vi "Check_Aero_Tunnel_on_Server.vi"(1 "Current Time":dbl format="%.2f", 2 "Ch Names":string[](array[string]), 3 "Values":dbl[](array[numeric]) format="%.2f") -> ()   [LabVIEW 2010]
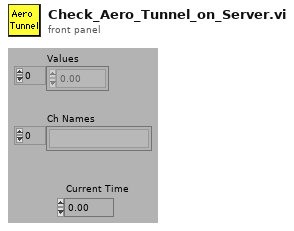
[diagram p1: front panel]
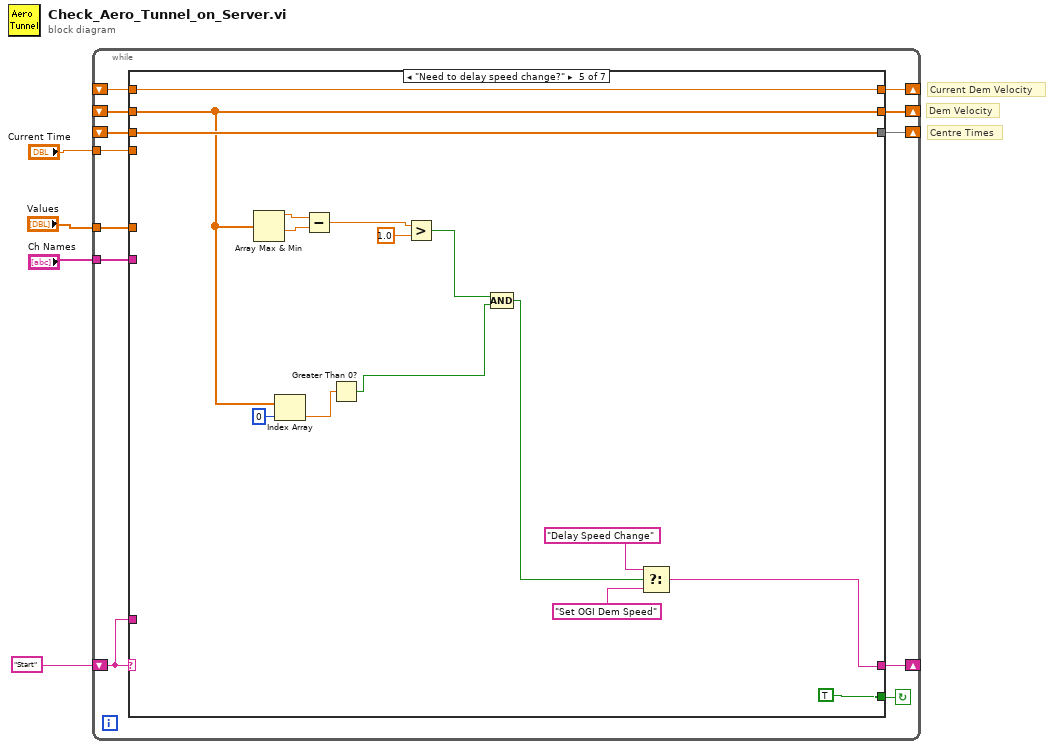
[diagram p0: block diagram]
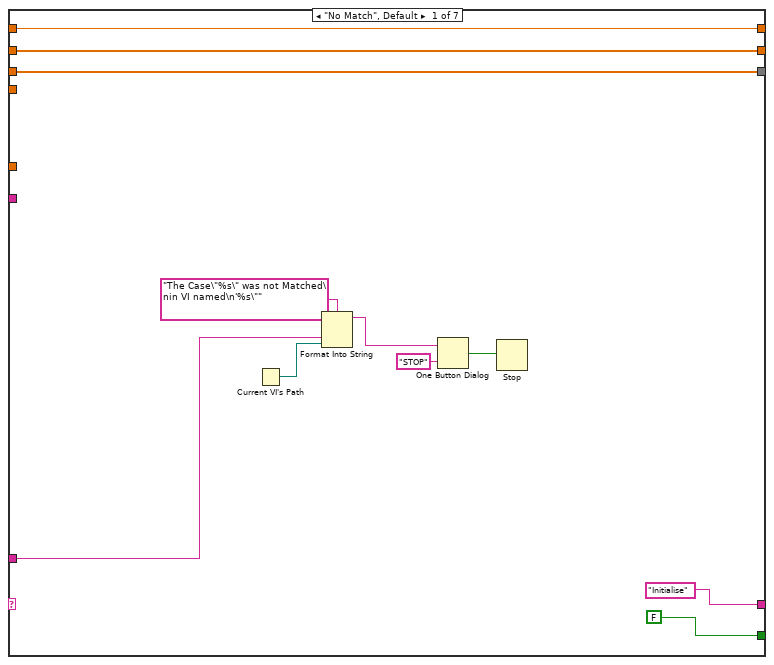
[diagram p2: hidden frame]
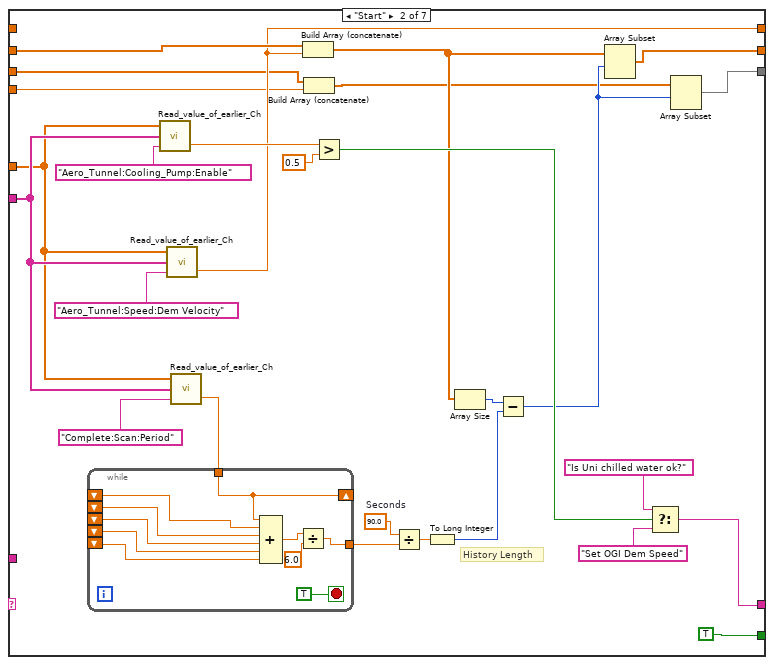
[diagram p3: hidden frame]
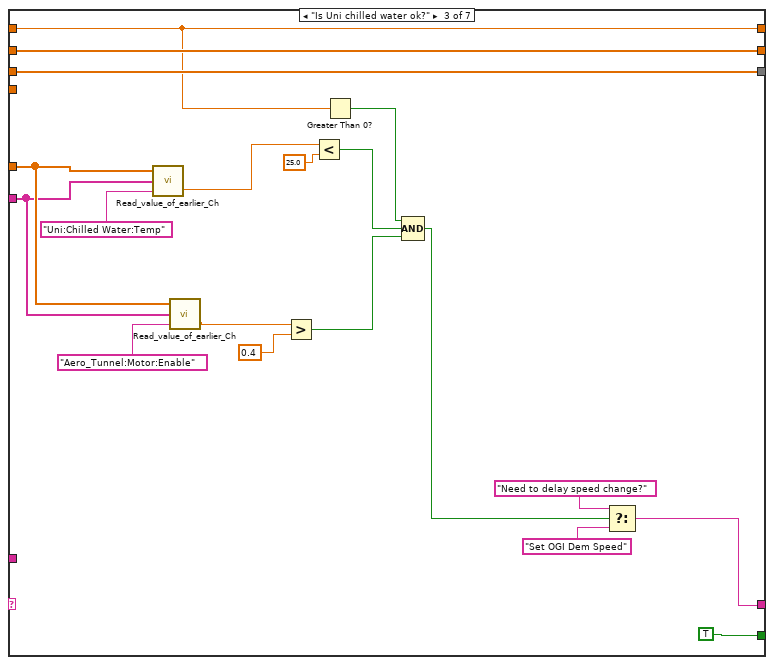
[diagram p4: hidden frame]
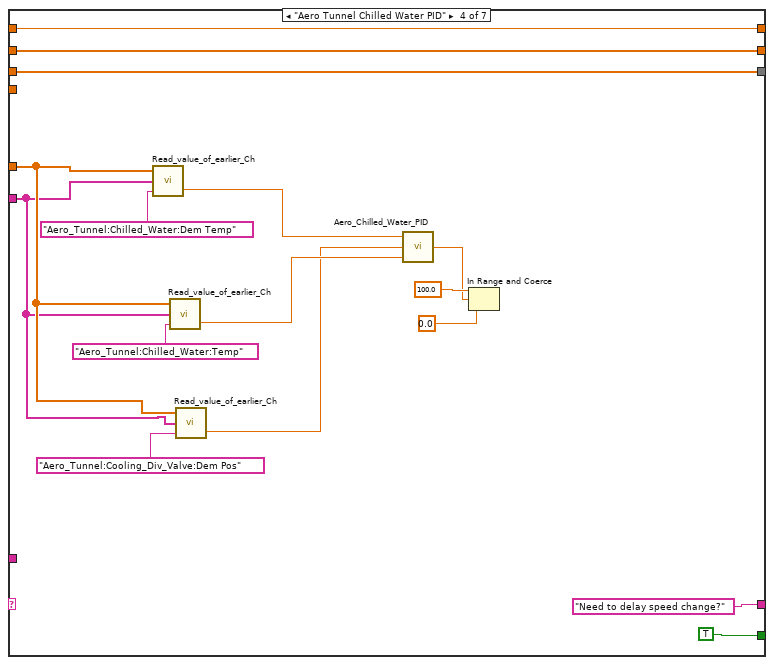
[diagram p5: hidden frame]
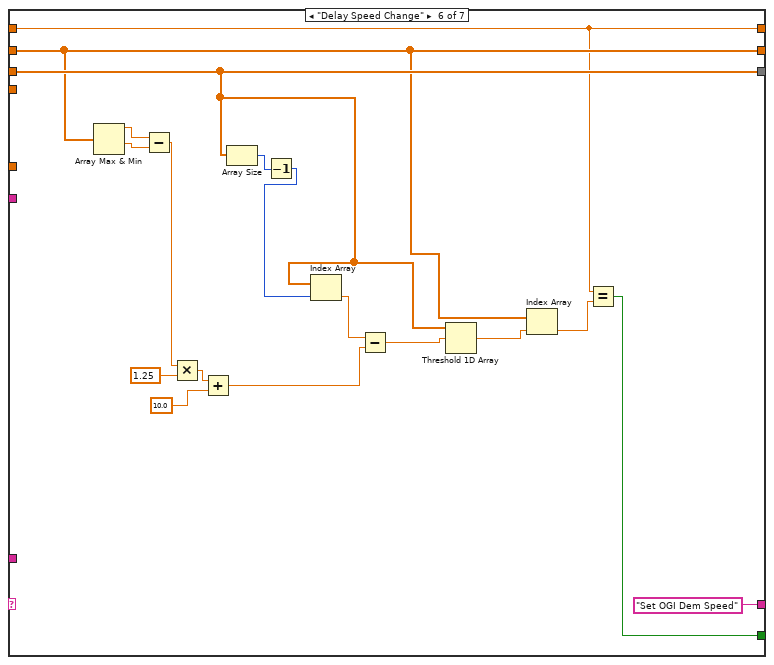
[diagram p6: hidden frame]
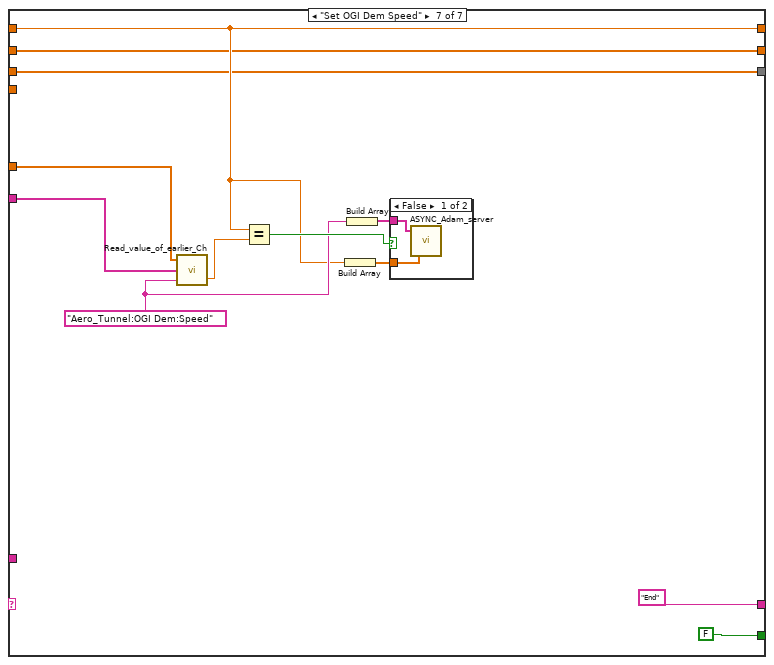
[diagram p7: hidden frame]
diagram:
  # "Dem Velocity"
  # "Centre Times"
  # "Current Dem Velocity"
  n1 = while {
    shift-left: "Start" -> [w14]
    shift-right: [w15] -> _
    tunnel: "Values" -> [w13]
    tunnel: "Ch Names" -> [w12]
    shift-right: [w11] -> _
    shift-left: _ -> [w10]
    shift-right: [w8] -> _
    shift-left: _ -> [w9]
    shift-right: [w5] -> _
    shift-left: _ -> [w6]
    tunnel: "Current Time" -> [w7]
    stop <- w16 continue-if-true
    n2 = case shown="\"Need to delay speed change?\"" w14 {
      tunnel: [FALSE TRUE TRUE TRUE TRUE w117 FALSE] -> w16
      tunnel: ["Initialise" w47 w78 "Need to delay speed change?" ("t") w113 "Set OGI Dem Speed" "End"] -> w15
      tunnel: w14 -> [w22 _ _ _ _ _ _]
      tunnel: w13 -> [_ w43 w73 w87 _ _ w143]
      tunnel: w12 -> [_ w44 w72 w86 _ _ w142]
      tunnel: [w19 w38 w67 w94 w107 w118 w136] -> w11
      tunnel: w10 -> [w19 _ w67 w94 w107 w118 w136]
      tunnel: w9 -> [w18 w39 w77 w97 w105 w119 w135]
      tunnel: [w18 w34 w77 w97 w105 w119 w135] -> w8
      tunnel: w7 -> [_ w31 _ _ _ _ _]
      tunnel: w6 -> [w17 w30 w76 w96 w112 w120 w134]
      tunnel: [w17 w28 w76 w96 w112 w120 w134] -> w5
      frame "No Match", Default {
        n3 = Current VI's Path() -> (path=w21:path)
        n4 = Format Into String(format string="The Case\"%s\" was not Matched\nin VI named\n'%s\"" ("Format String"), w22, w21) -> (resulting string=w25:string)  [unwired: 2 in, 1 out]
        n5 = One Button Dialog(message=w25, button name ("OK")="STOP") -> (true=w23:bool)
        n6 = Stop(stop? (T)=w23) -> ()
      }
      frame "Start" {
        w40 = 90.0  # Seconds
        # "History Length"
        n7 = call "Read_value_of_earlier_Ch.vi"("Desired Ch to Read"="Aero_Tunnel:Cooling_Pump:Enable", "Ch names"=w44, "Present scan array"=w43) -> ("Value"=w51:dbl)  [unwired: 1 in, 1 out]
        n8 = call "Read_value_of_earlier_Ch.vi"("Desired Ch to Read"="Aero_Tunnel:Speed:Dem Velocity", "Ch names"=w44, "Present scan array"=w43) -> ("Value"=w38:dbl)  [unwired: 1 in, 1 out]
        n9 = call "Read_value_of_earlier_Ch.vi"("Desired Ch to Read"="Complete:Scan:Period", "Ch names"=w44, "Present scan array"=w43) -> ("Value"=w42:dbl)  [unwired: 1 in, 1 out]
        n10 = while {
          shift-right: [w64] -> _
          shift-left: _ -> [w63]
          tunnel: w42 -> [w64]
          shift-left: _ -> [w62]
          shift-left: _ -> [w61]
          shift-left: _ -> [w60]
          shift-left: _ -> [w59]
          tunnel: [w55] -> w41
          stop <- TRUE stop-if-true
          n11 = Compound Arithmetic op=ADD(w64, w63, w62, w61, w60, w59) -> (w57:dbl)
          n12 = Divide(x=w57, y=6.0) -> (x/y=w55:dbl)
        }
        n13 = Build Array (concatenate)(w39, w38) -> (w32:dbl[])
        n14 = Build Array (concatenate)(w30, w31) -> (w29:dbl[])
        n15 = Greater?(x=w51, y=0.5) -> (0:w49:bool)
        n16 = Divide(x=w40, y=w41) -> (x/y=w36:dbl)
        n17 = To Long Integer(number=w36) -> (32bit integer=w35:i32)
        n18 = Array Size(array=w32) -> (size(s)=w37:i32)
        n19 = Subtract(x=w37, y=w35) -> (x-y=w33:i32)
        n20 = Array Subset(array=w32, index=w33) -> (w34:dbl[])  [unwired: 1 in]
        n21 = Select(t="Is Uni chilled water ok?", s=w49, f="Set OGI Dem Speed") -> (s? t:f=w47:string)
        n22 = Array Subset(array=w29, index=w33) -> (w28:dbl[])  [unwired: 1 in]
      }
      frame "Is Uni chilled water ok?" {
        n23 = call "Read_value_of_earlier_Ch.vi"("Desired Ch to Read"="Uni:Chilled Water:Temp", "Ch names"=w72, "Present scan array"=w73) -> ("Value"=w81:dbl)  [unwired: 1 in, 1 out]
        n24 = call "Read_value_of_earlier_Ch.vi"("Desired Ch to Read"="Aero_Tunnel:Motor:Enable", "Ch names"=w72, "Present scan array"=w73) -> ("Value"=w70:dbl)  [unwired: 1 in, 1 out]
        n25 = Greater?(x=w70, y=0.4) -> (0:w68:bool)
        n26 = Less?(x=w81, y=25.0) -> (x < y?=w69:bool)
        n27 = Greater Than 0?(x=w67) -> (x > 0?=w66:bool)
        n28 = Compound Arithmetic op=AND(w66, w69, w68) -> (w65:bool)
        n29 = Select(t="Need to delay speed change?", s=w65, f="Set OGI Dem Speed") -> (s? t:f=w78:string)
      }
      frame "Aero Tunnel Chilled Water PID" {
        n30 = call "Read_value_of_earlier_Ch.vi"("Desired Ch to Read"="Aero_Tunnel:Chilled_Water:Dem Temp", "Ch names"=w86, "Present scan array"=w87) -> ("Value"=w90:dbl)  [unwired: 1 in, 1 out]
        n31 = call "Read_value_of_earlier_Ch.vi"("Desired Ch to Read"="Aero_Tunnel:Chilled_Water:Temp", "Ch names"=w86, "Present scan array"=w87) -> ("Value"=w89:dbl)  [unwired: 1 in, 1 out]
        n32 = call "Read_value_of_earlier_Ch.vi"("Desired Ch to Read"="Aero_Tunnel:Cooling_Div_Valve:Dem Pos", "Ch names"=w86, "Present scan array"=w87) -> ("Value"=w85:dbl)  [unwired: 1 in, 1 out]
        n33 = call "Aero_Chilled_Water_PID.vi"("Present Value"=w89, "Previous Control Sum"=w85, "Setpoint"=w90) -> ("Dem Output"=w91:dbl)
        n34 = In Range and Coerce(upper limit=100.0, x=w91, lower limit=0.0) -> ()  [unwired: 2 out]
      }
      frame "Need to delay speed change?" {
        n35 = Array Max & Min(array=w105) -> (max value=w110:dbl, min value=w111:dbl)  [unwired: 2 out]
        n36 = Index Array(array=w105, index=0) -> (element=w104:dbl)
        n37 = Subtract(x=w110, y=w111) -> (x-y=w108:dbl)
        n38 = Greater Than 0?(x=w104) -> (x > 0?=w102:bool)
        n39 = Greater?(x=w108, y=1.0) -> (0:w103:bool)
        n40 = Compound Arithmetic op=AND(w103, w102) -> (w100:bool)
        n41 = Select(t="Delay Speed Change", s=w100, f="Set OGI Dem Speed") -> (s? t:f=w113:string)
      }
      frame "Delay Speed Change" {
        n42 = Array Max & Min(array=w119) -> (max value=w132:dbl, min value=w133:dbl)  [unwired: 2 out]
        n43 = Subtract(x=w132, y=w133) -> (x-y=w123:dbl)
        n44 = Multiply(x=w123, y=1.25) -> (x*y=w125:dbl)
        n45 = Add(x=w125, y=10.0) -> (x+y=w128:dbl)
        n46 = Array Size(array=w120) -> (size(s)=w122:i32)
        n47 = Decrement(x=w122) -> (x-1=w121:i32)
        n48 = Index Array(array=w120, index=w121) -> (element=w127:dbl)
        n49 = Subtract(x=w127, y=w128) -> (x-y=w129:dbl)
        n50 = Threshold 1D Array(2:w129, 3:w120) -> (0:w130:dbl)  [unwired: 1 out]
        n51 = Index Array(array=w119, index=w130) -> (element=w131:dbl)
        n52 = Equal?(x=w118, y=w131) -> (x = y?=w117:bool)
      }
      frame "Set OGI Dem Speed" {
        w139 = "Aero_Tunnel:OGI Dem:Speed"
        n53 = call "Read_value_of_earlier_Ch.vi"("Desired Ch to Read"=w139, "Ch names"=w142, "Present scan array"=w143) -> ("Value"=w141:dbl)  [unwired: 1 in, 1 out]
        n54 = Equal?(x=w136, y=w141) -> (x = y?=w140:bool)
        n55 = Build Array(w136) -> (w137:dbl[])
        n56 = Build Array(w139) -> (w138:string[])
        n57 = case shown="False" w140 {
          tunnel: w137 -> [w147 _]
          tunnel: w138 -> [w146 _]
          frame False {
            n58 = call "ASYNC_Adam_server.vi"("Values"=w147, "Channel Names"=w146) -> ()  [unwired: 1 in, 3 out]
          }
          frame True {
          }
        }
      }
    }
  }
